vi "Test - LM 79 stabilization.vi"() -> ()   [LabVIEW 2013]
uses:
  Controls/Stabilization.ctl
  <vilib>/Utility/file.llb/Read From Spreadsheet File (DBL).vi
panel:
  out "Stabilization Data":T1
  out "Boolean":bool
  out "size(s)":i32
  out "Array":dbl[](array[numeric])
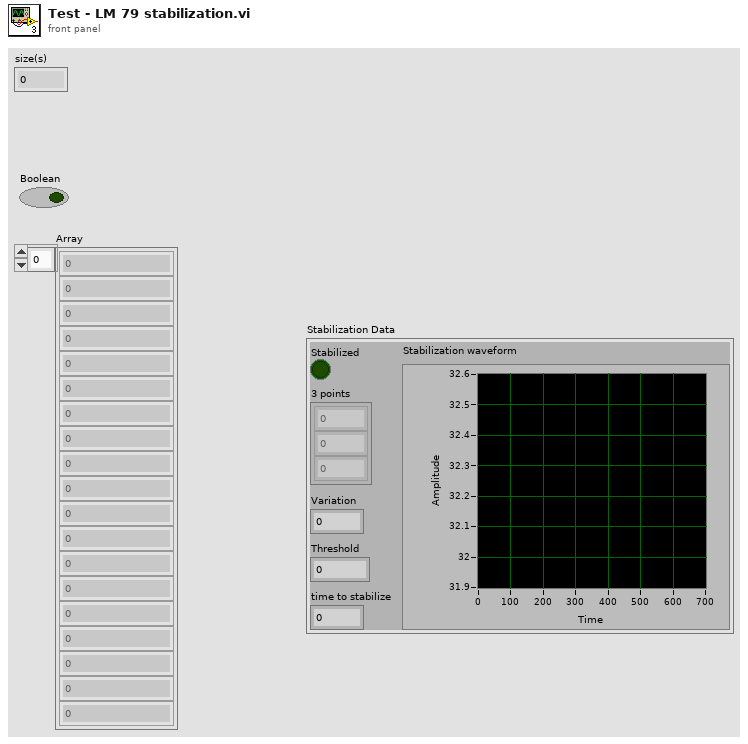
[diagram p1: front panel]
types:
  T1 = typedef "Stabilization.ctl" = cluster{"Stabilization waveform":waveform(dbl), "Variation":dbl, "Stabilized":bool, "Threshold":dbl, "time to stabilize":dbl, "3 points":dbl[]}
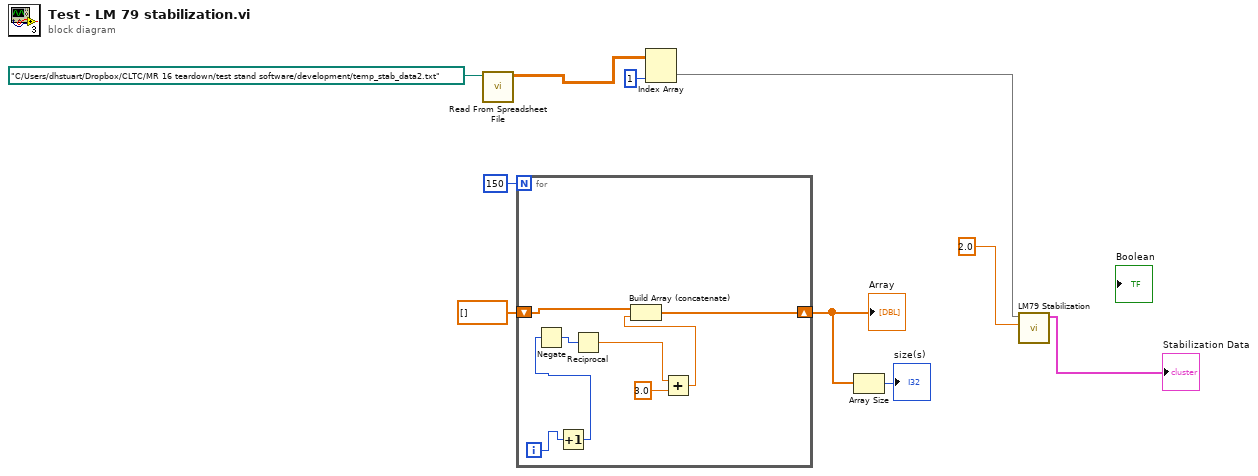
[diagram p0: block diagram]
diagram:
  n1 = call-poly <vilib>:"Read From Spreadsheet File.vi"("file path (dialog if empty)"=path "C:/Users/dhstuart/Dropbox/CLTC/MR 16 teardown/test stand software/development/temp_stab_data2.txt") -> ("all rows"=w4:dbl[][])  [unwired: 6 in, 4 out]
  n2 = for {
    N: 150 -> [_]
    shift-right: [w18] -> w5
    shift-left: dbl[] [] -> [w17]
    i -> [w16]
    n3 = Increment(x=w16) -> (x+1=w14:i32)
    n4 = Negate(x=w14) -> (-x=w15:i32)
    n5 = Reciprocal(x=w15) -> (1/x=w13:dbl)
    n6 = Add(x=w13, y=3.0) -> (x+y=w11:dbl)
    n7 = Build Array (concatenate)(w17, w11) -> (w18:dbl[])
  }
  "Array" <- w5
  n8 = Index Array(array=w4, index (col)=1 ("disabled index (col)")) -> (element=w2:dbl[])  [unwired: 1 in]
  n9 = Array Size(array=w5) -> (size(s)=→"size(s)":i32)
  n10 = call "LM79 Stabilization.vi"("Time Between\nMeasurements (ms)"=2.0 ("dt (ms)"), "Data over time"=w2) -> ("Stabilization Data"=→"Stabilization Data":T1)  [unwired: 8 in, 1 out]
